vi "Set Temp Ramp Rate--Method.vi"(8 "error in (no error)":errorcluster, 10 "Temp Ramp Data":T1, 11 "Watlow F4T in":refnum<class "Watlow F4T.lvclass">) -> (0 "error out":errorcluster, 3 "Watlow F4T out":refnum<class "Watlow F4T.lvclass">)   [LabVIEW 2024, in "Watlow F4T.lvclass"]
uses:
  Watlow F4T.lvclass
  Process Controller/Controls/Temp Ramp Rate Data--Cluster.ctl
  Process Controller/Controls/Temperature Units--Enum.ctl
  Process Controller/Controls/Rate Units--Enum.ctl
  Process Controller/_Thermal Process Controller.lvclass
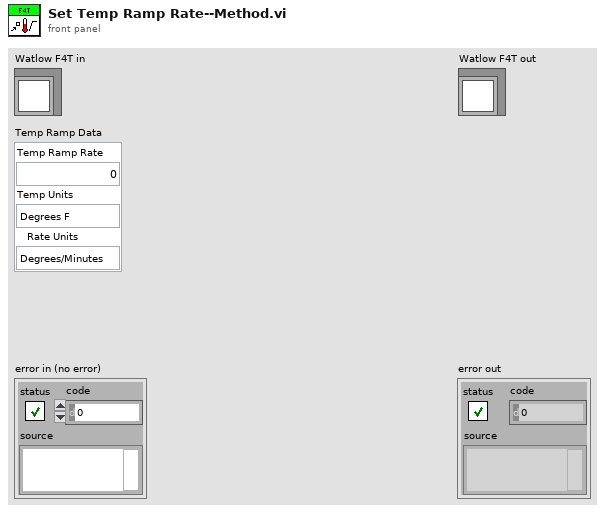
[diagram p1: front panel]
types:
  T1 = typedef "_Thermal Process Controller.lvclass/Temp Ramp Rate Data--Cluster.ctl" = cluster{"Temp Ramp Rate":dbl, "Temp Units":T2, "Rate Units":T3}
  T2 = typedef "_Thermal Process Controller.lvclass/Temperature Units--Enum.ctl" = enum16{"Degrees F", "Degrees C", "Degrees K"}
  T3 = typedef "_Thermal Process Controller.lvclass/Rate Units--Enum.ctl" = enum16{"Degrees/Minutes", "Degrees/Hours"}
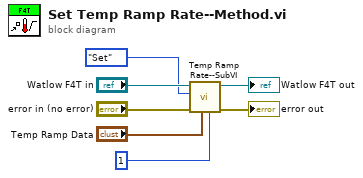
[diagram p0: block diagram]
diagram:
  n1 = call "Temp Ramp Rate--SubVI.vi"("Instance(1)"=1, "Temp Ramp Data"="Temp Ramp Data", "error in (no error)"="error in (no error)", "Get/Set"=enum16{"Get", "Set"}."Set", "Watlow F4T in"="Watlow F4T in") -> ("error out"=→"error out":errorcluster, "Watlow F4T out"=→"Watlow F4T out":refnum<class "Watlow F4T.lvclass">)  [unwired: 4 in, 1 out]
